vi "camara 3.vi"() -> ()   [LabVIEW 2010]
uses:
  <vilib>/addons/PixeLINK/Low Level Functions/CAMERA_FEATURES.llb/TDPU-CameraFeatures-PixelFormat.ctl
  <vilib>/Utility/error.llb/DialogType.ctl
  <vilib>/vision/Image Controls.llb/IMAQ Image.ctl
  <vilib>/addons/PixeLINK/Low Level Functions/ACQUISITION.llb/TDPU-Acquisition-StreamState.ctl
  <vilib>/addons/PixeLINK/Low Level Functions/CAMERA_FEATURES.llb/TDPU-CameraFeatures-FeatureFlags.ctl
  <vilib>/addons/PixeLINK/Low Level Functions/CAMERA_FEATURES.llb/TDPU-CameraFeatures-FeatureIds.ctl
  <vilib>/DAQmx/create/channels.llb/DAQmx Create Channel (AO-Voltage-Basic).vi
  <vilib>/DAQmx/configure/timing.llb/DAQmx Timing (Use Waveform).vi
panel:
  in  "DAQ Fs (S/s)":dbl=10000.0
  in  "Maximum Value":dbl=10.0 format="%0.2f"
  in  "Minimum Value":dbl=-10.0 format="%0.2f"
  in  "Physical Channel":tag="Dev1/ao0"
  in  "Tab Control":enum32{"Camara", "Control"}(tab)
  in  "Pixel Format Requerido":T1 items=["PIXEL_FORMAT_MONO8", "PIXEL_FORMAT_MONO16", "PIXEL_FORMAT_YUV422", "PIXEL_FORMAT_BAYER8_GRBG", "PIXEL_FORMAT_BAYER16_GRBG", "PIXEL_FORMAT_RGB24", "PIXEL_FORMAT_RGB48", "PIXEL_FORMAT_BAYER8_RGGB", "PIXEL_FORMAT_BAYER8_GBRG ", "PIXEL_FORMAT_BAYER8_BGGR ", "PIXEL_FORMAT_BAYER16_RGGB ", "PIXEL_FORMAT_BAYER16_GBRG", "PIXEL_FORMAT_BAYER16_BGGR", "PIXEL_FORMAT_RGB32"]
  in  "Exposure Time (ms)":dbl(slide) scale=0.1..2000.0
  in  "Gain":dbl(slide) scale=0.0..25.0
  in  "Red":sgl(slide) scale=0.0..4.0
  in  "Green":sgl(slide) scale=0.0..4.0
  in  "Blue":sgl(slide) scale=0.0..4.0
  in  "Selector":u16(ring) items=["776002034"]
  out "Numero de Camaras":u32
  in  "Camara ON?":bool
  in  "Ajuste ON?":bool=TRUE
  in  "Control ON?":bool=TRUE
  in  "Reset Control":bool
  in  "Parametros Ajuste nm2freq":cluster{"Cruce por cero":dbl, "Pendiente":dbl}={"Cruce por cero"=0.04, "Pendiente"=0.0031}
  in  "Frecuencia":dbl=2000.0
  in  "lamda (nm)":dbl=546.1
  out "Contraste":dbl(graph)
  out "Señal de Control":cluster{dbl[], "Señal de Control":dbl[]}(graph)
  out "Waveform":waveform(dbl)(graph)
  out "Image":T2(plugin-control)
  in  "Stop App":bool
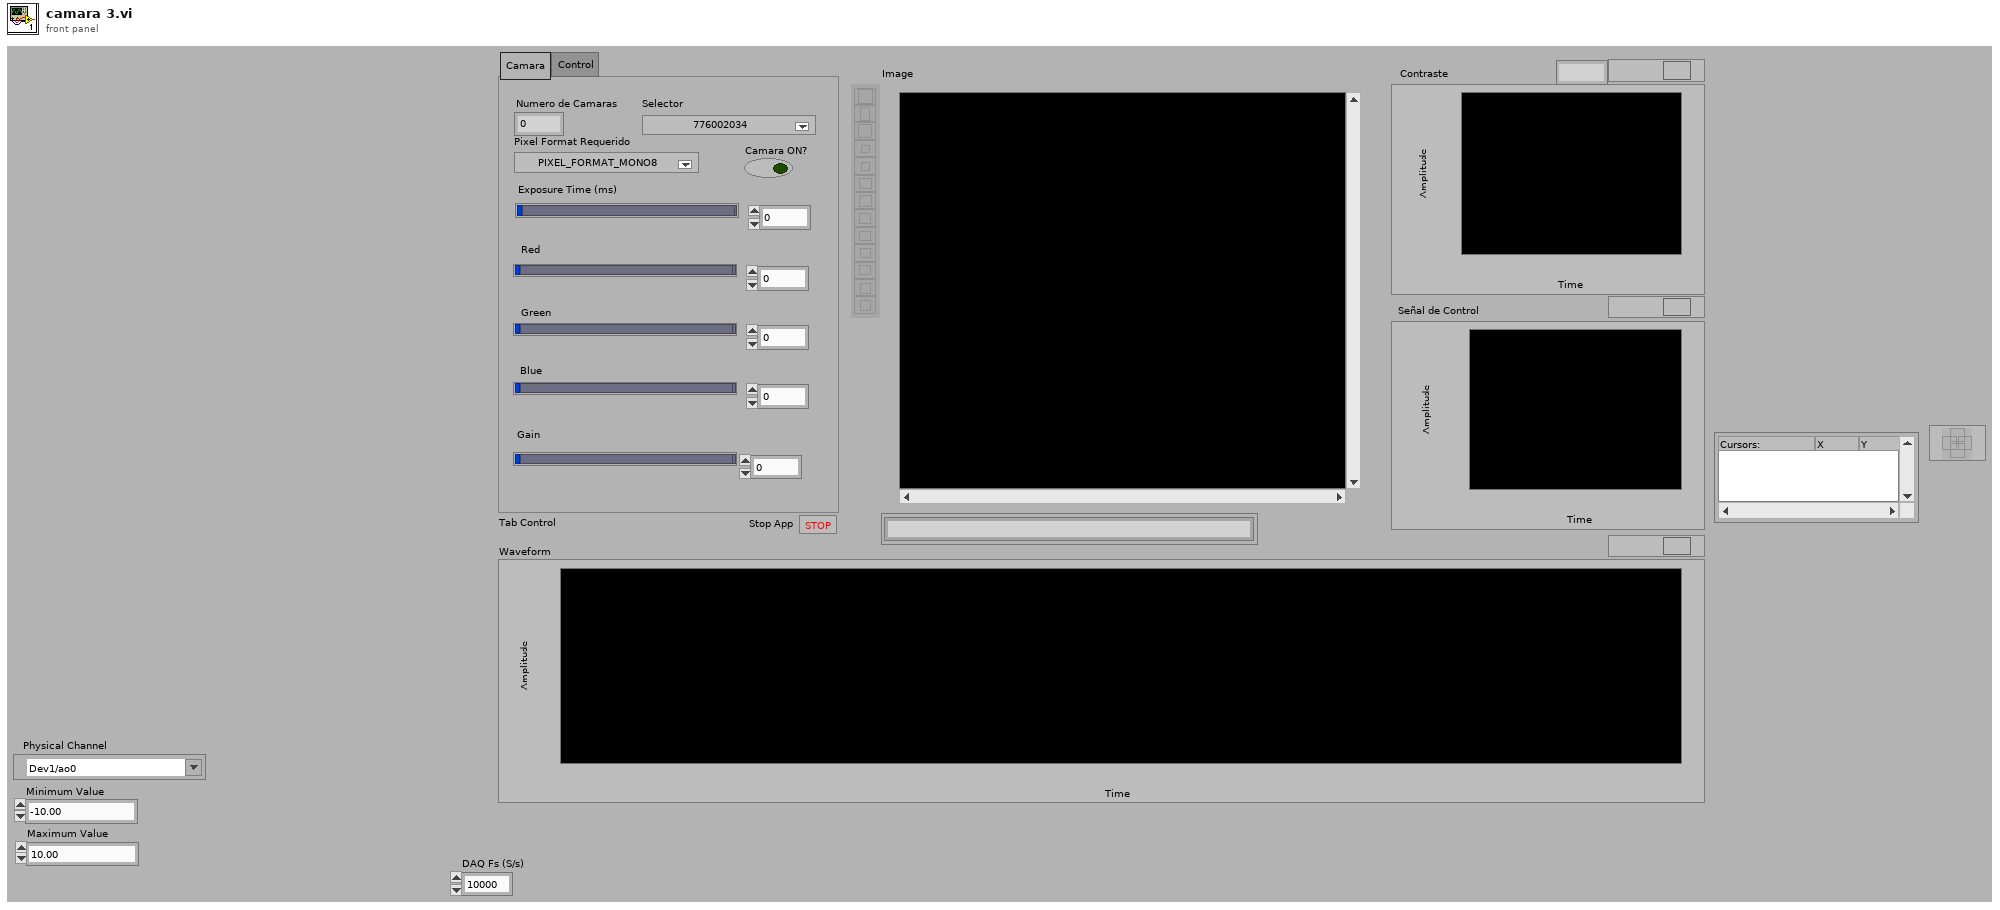
[diagram p1: front panel]
types:
  T1 = typedef "TDPU-CameraFeatures-PixelFormat.ctl" = u16
  T2 = typedef "IMAQ Image.ctl" = refnum<image>
  T3 = cluster{"DAQ Fs (S/s)":dbl, "task":refnum<k21>, "error":errorcluster}
  T4 = cluster{"lamda (nm)":dbl, "Base frecuency":dbl, "Parametros Ajuste nm2freq":cluster{"Cruce por cero":dbl, "Pendiente":dbl}}
  T5 = cluster{"Amplitud":dbl, "Media":dbl, "Sigma":dbl}
  T6 = cluster{"hCamera":u32, "errorCamera":errorcluster}
  T7 = typedef "DialogType.ctl" = u16
  T8 = typedef "Image Type" = u32
  T9 = typedef "TDPU-Acquisition-StreamState.ctl" = u32
  T10 = typedef "TDPU-CameraFeatures-FeatureIds.ctl" = u32
  T11 = typedef "TDPU-CameraFeatures-FeatureFlags.ctl" = u32
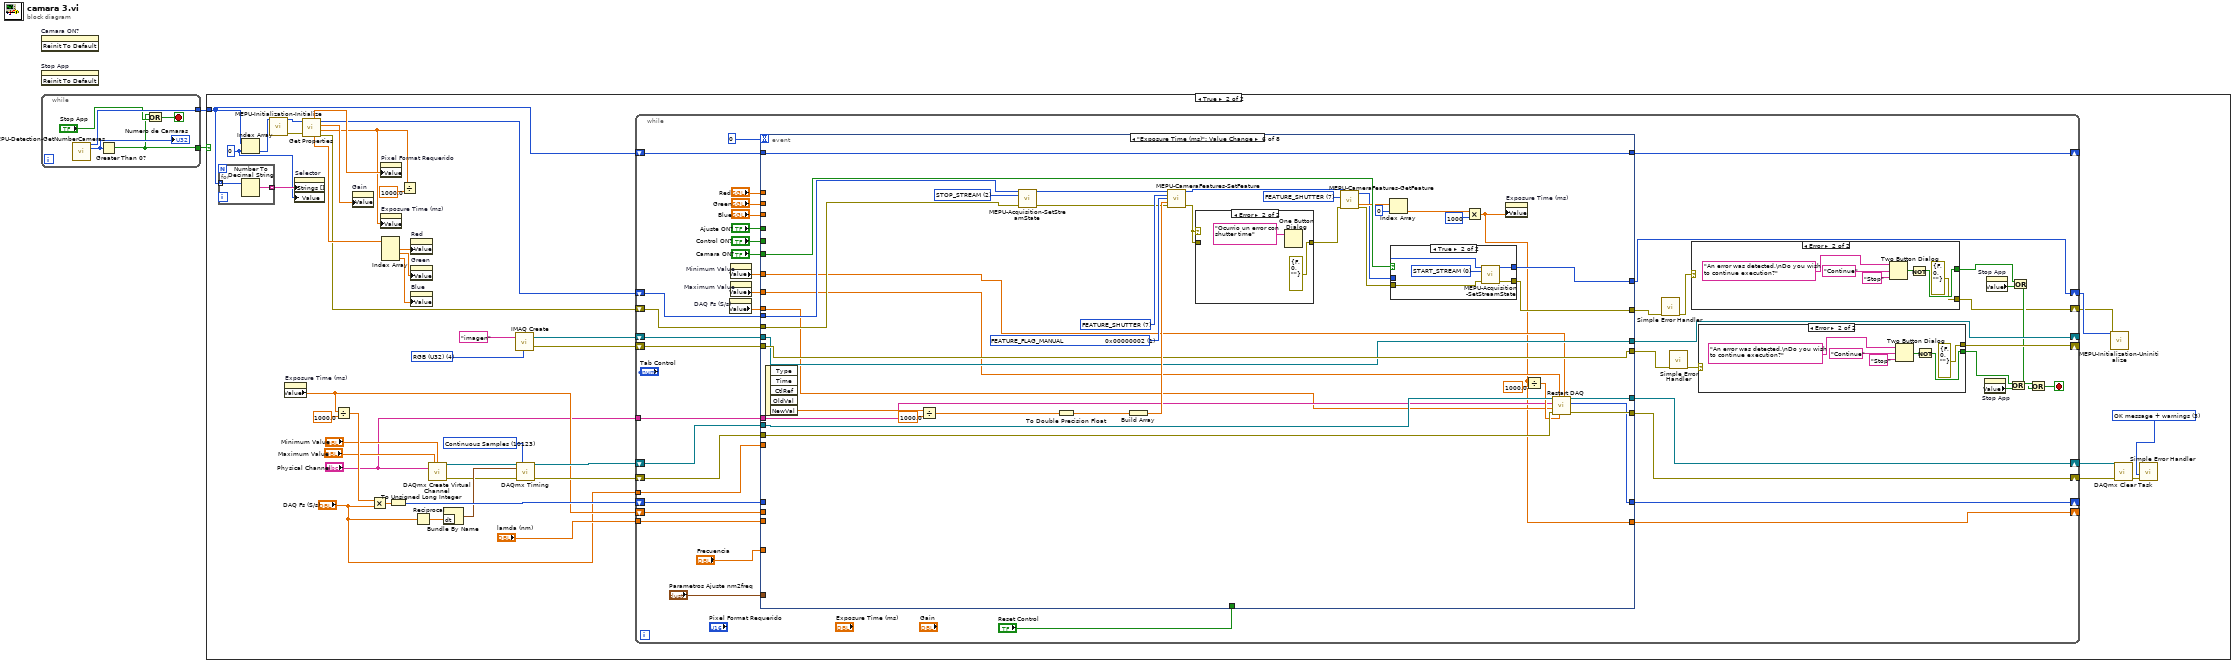
[diagram p0: block diagram]
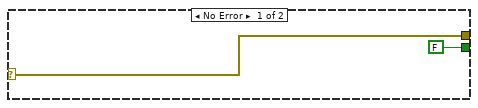
[diagram p3: hidden frame]
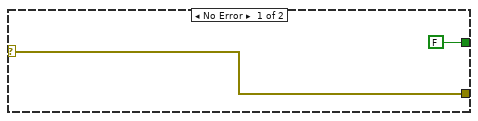
[diagram p4: hidden frame]
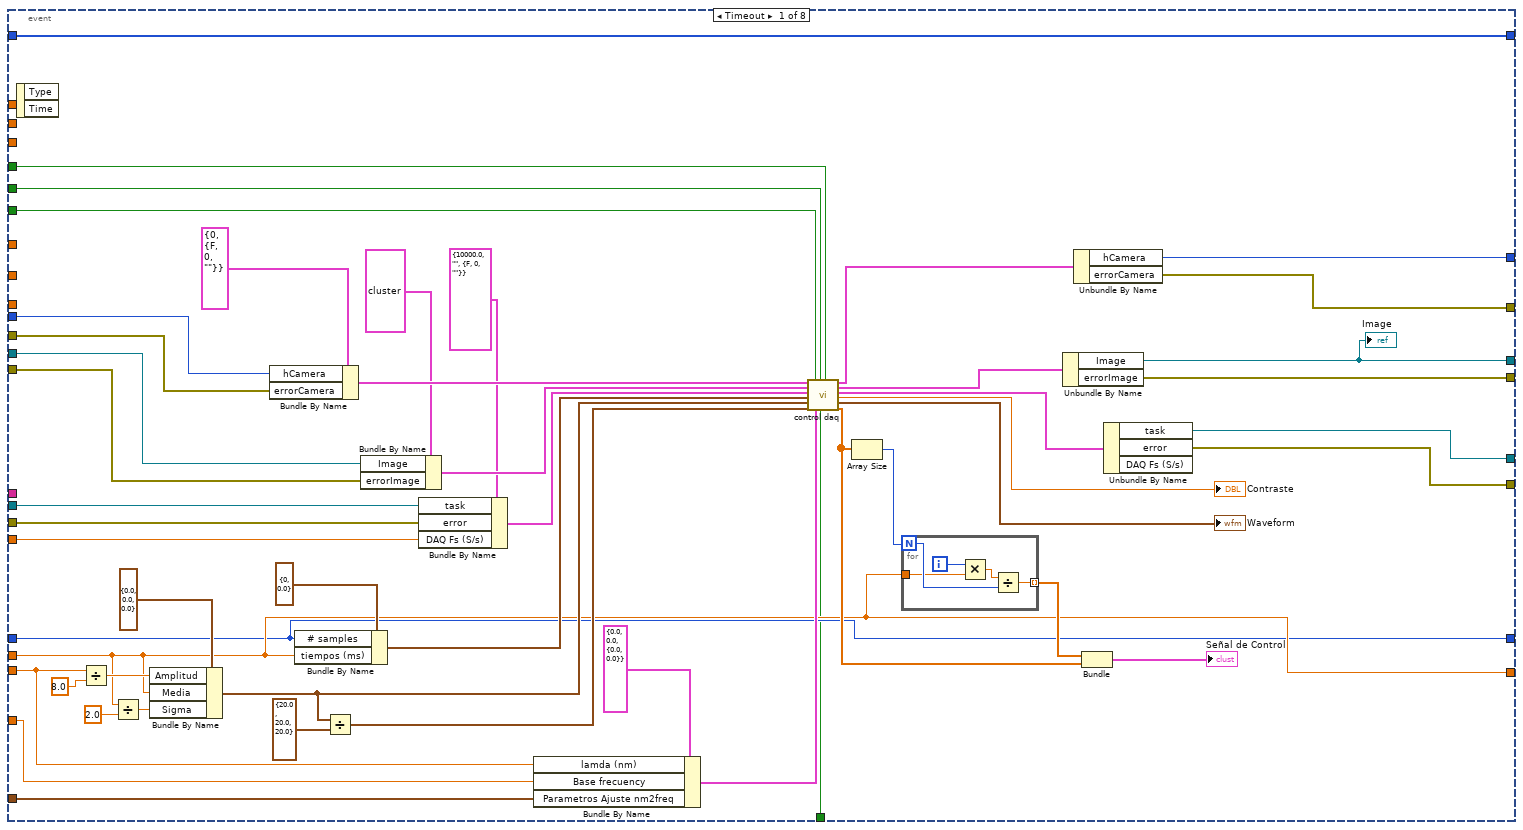
[diagram p5: hidden frame]
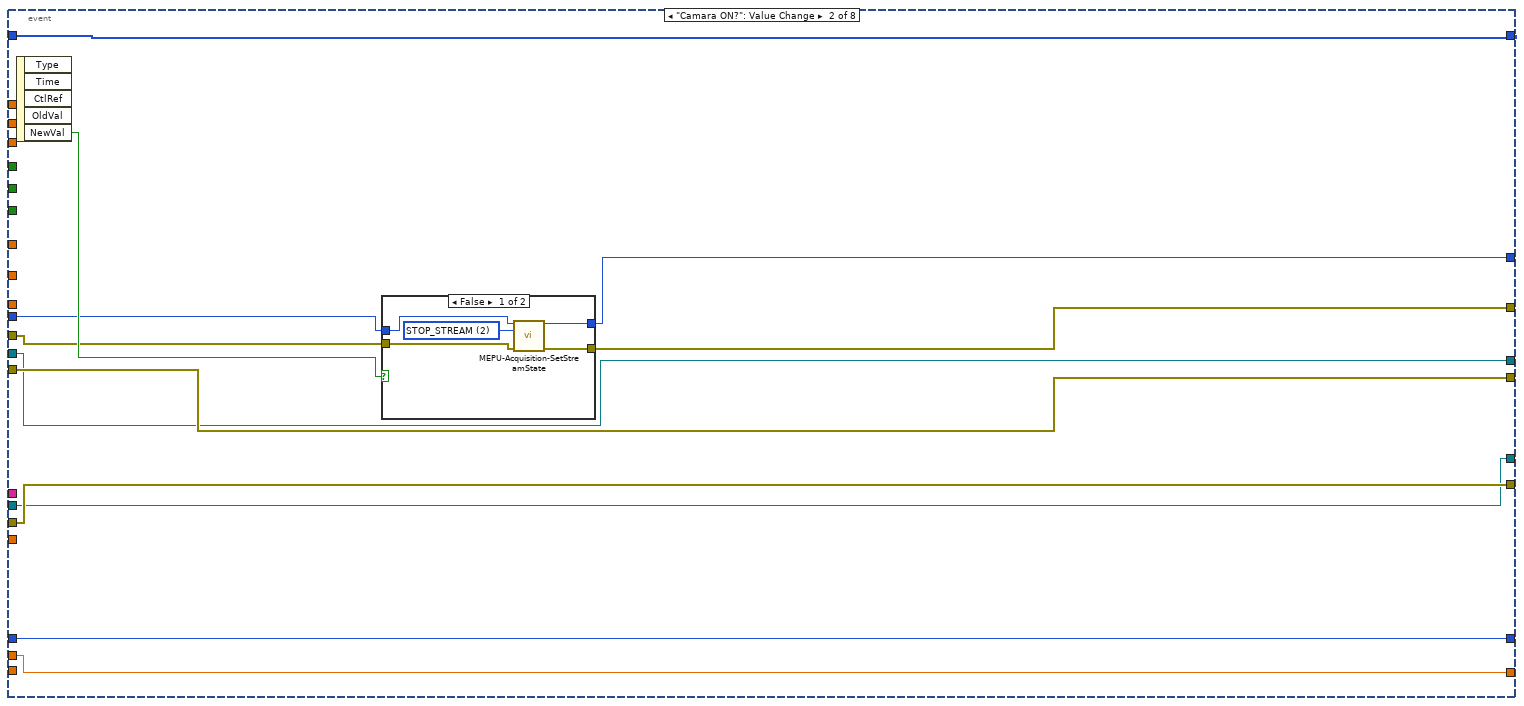
[diagram p6: hidden frame]
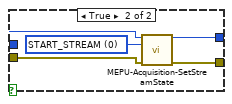
[diagram p7: hidden frame]
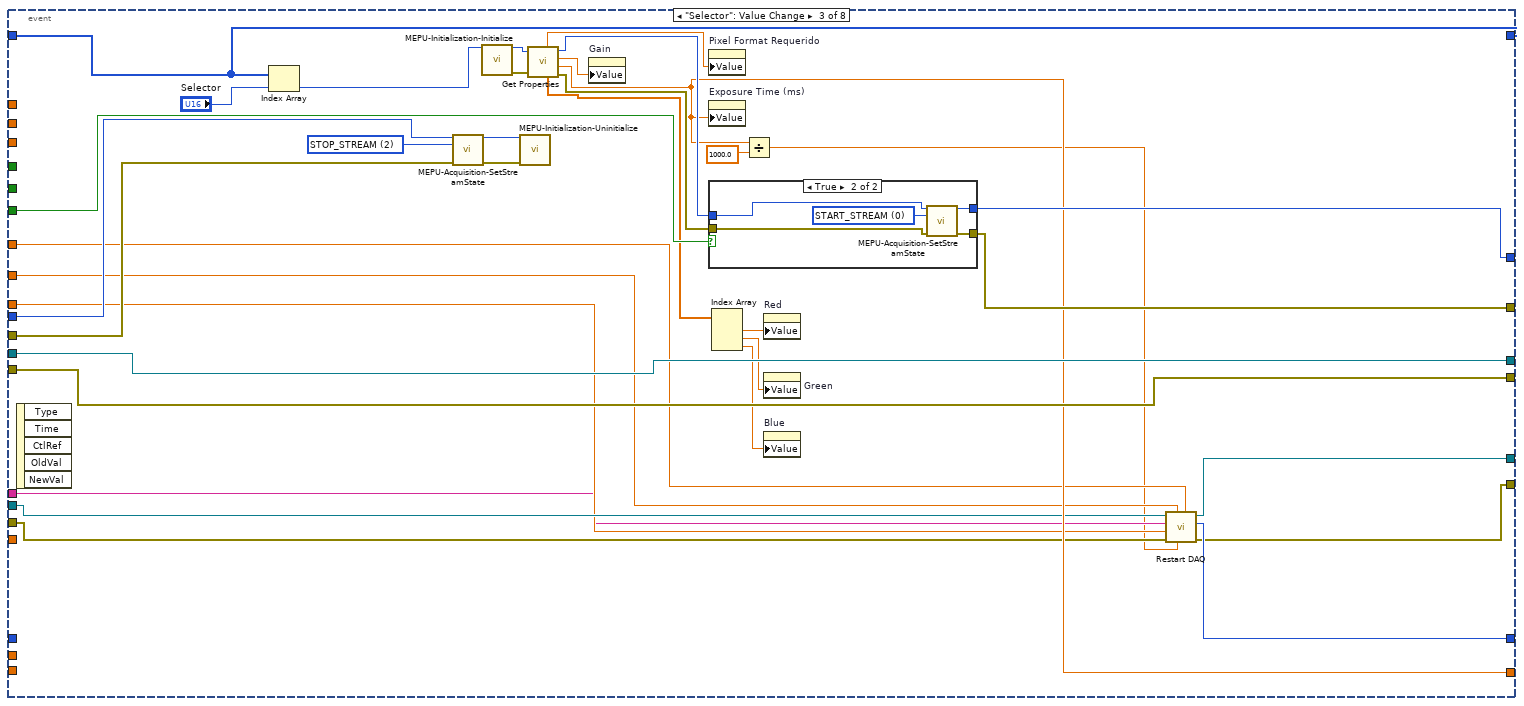
[diagram p8: hidden frame]
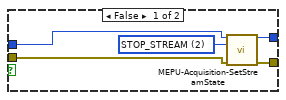
[diagram p9: hidden frame]
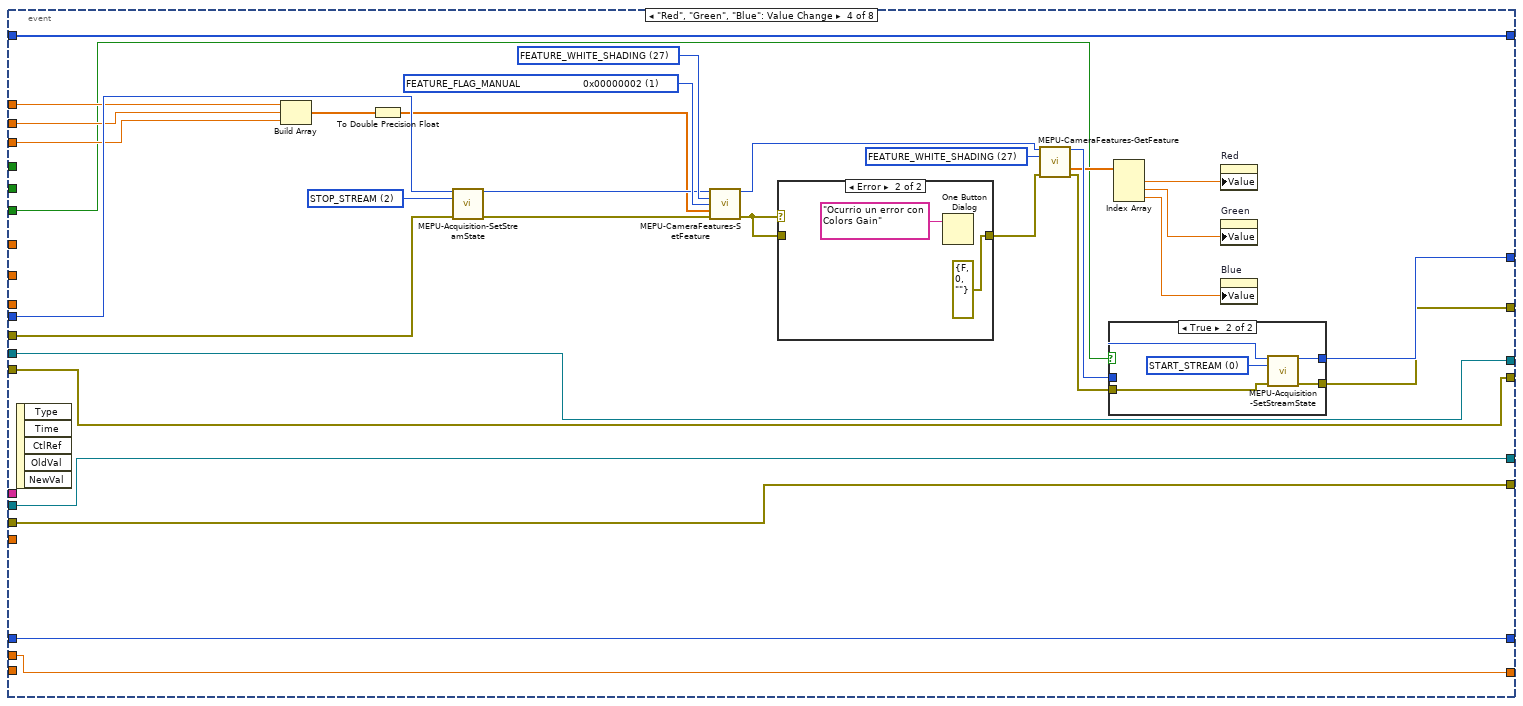
[diagram p10: hidden frame]
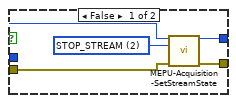
[diagram p11: hidden frame]
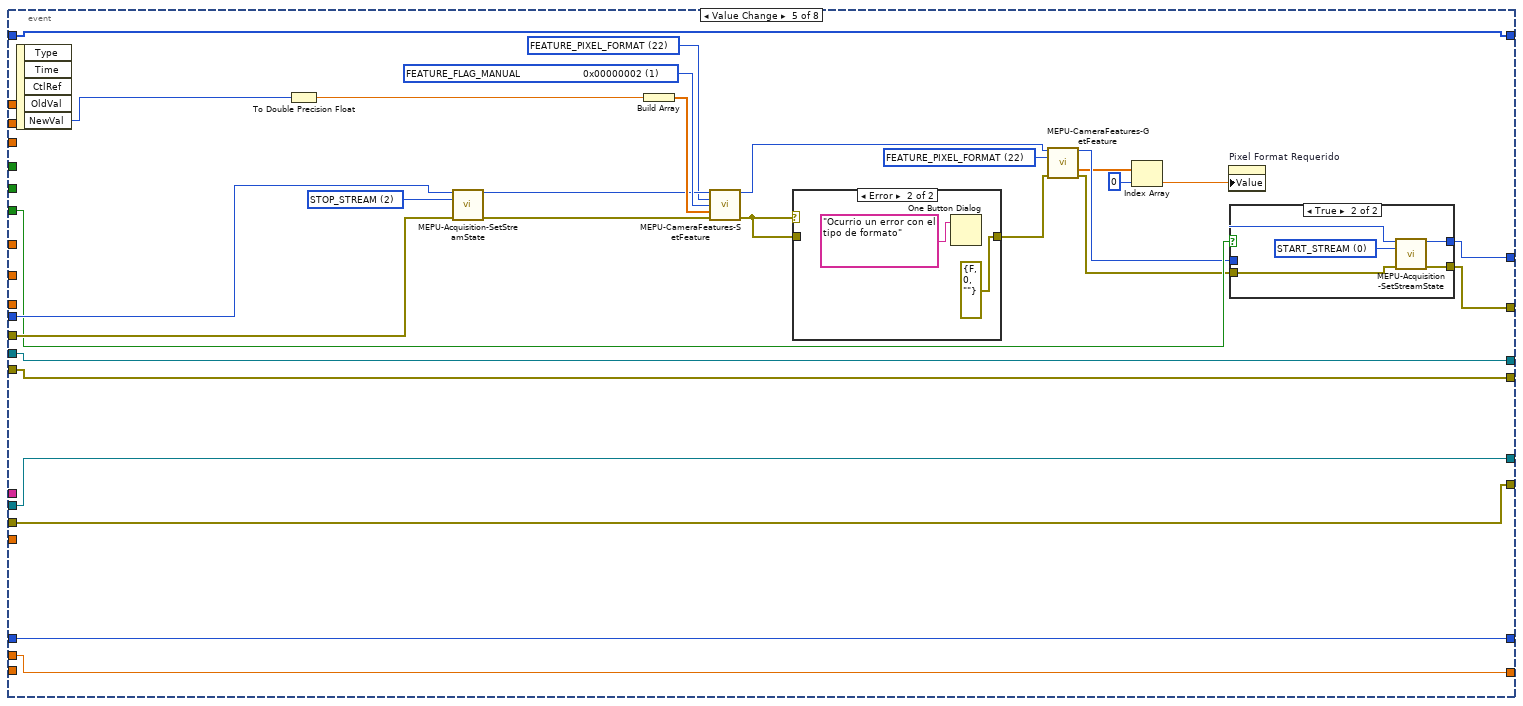
[diagram p13: hidden frame]
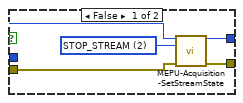
[diagram p14: hidden frame]
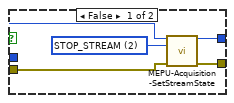
[diagram p16: hidden frame]
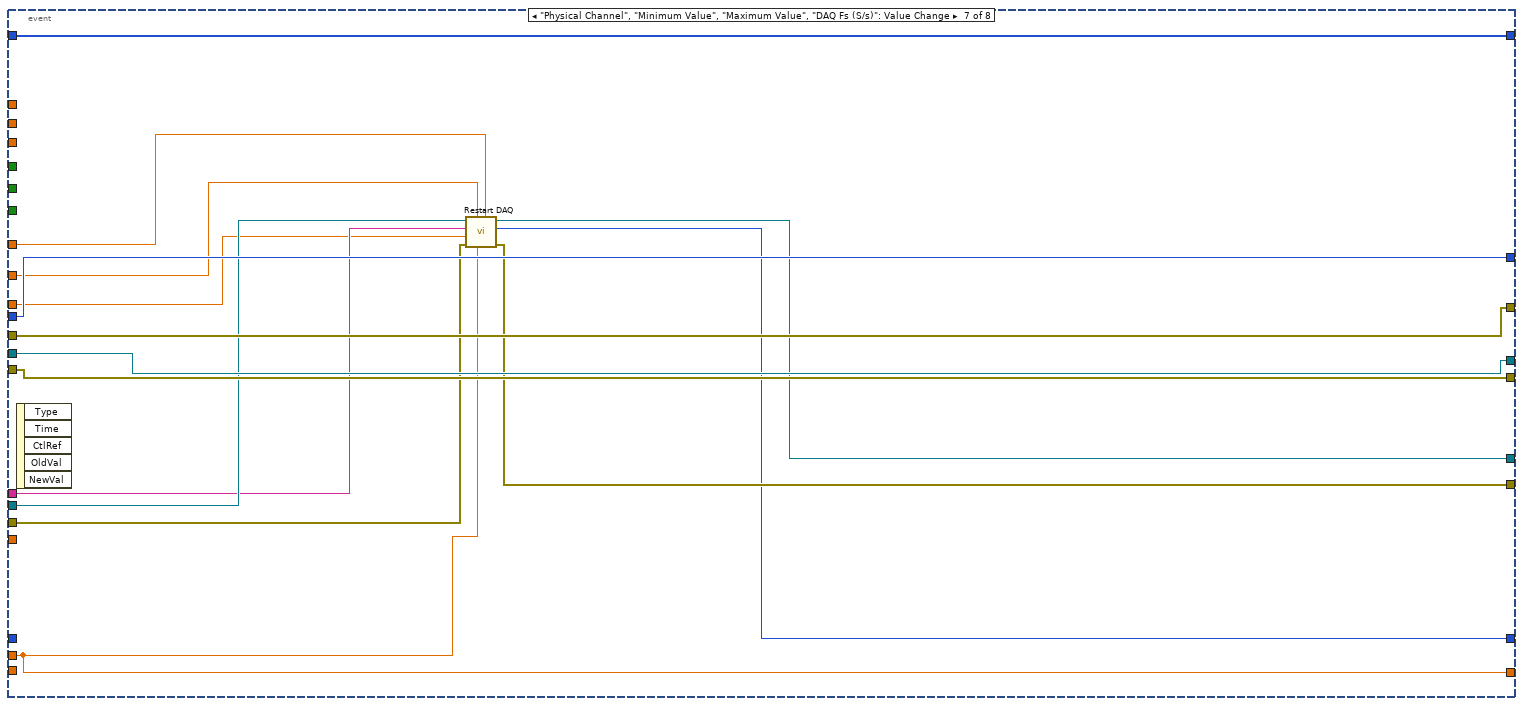
[diagram p18: hidden frame]
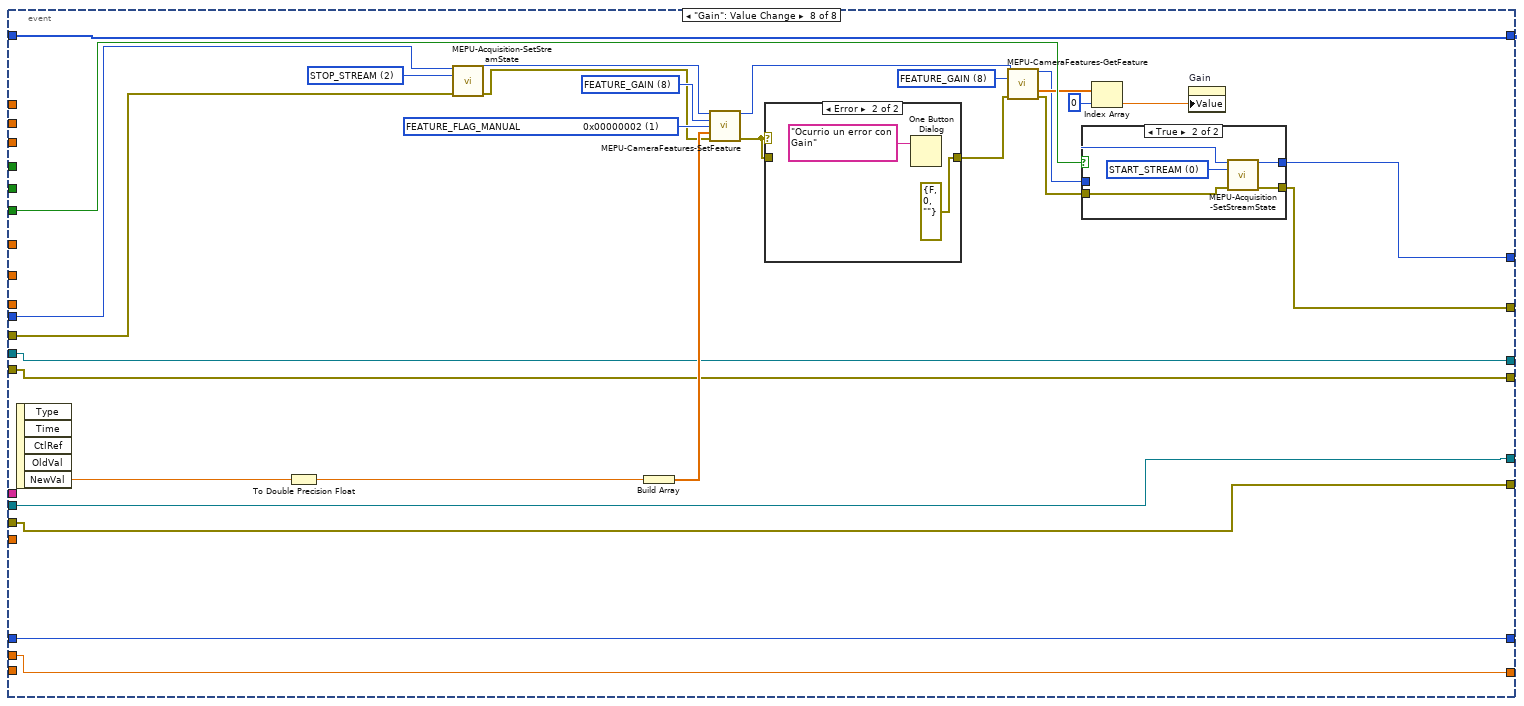
[diagram p19: hidden frame]
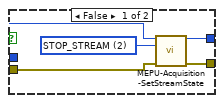
[diagram p20: hidden frame]
diagram:
  n1 = invoke on="Camara ON?" class="Bool (strict)" method="Reinit To Default"() -> ()  [unwired: 3 in, 3 out]
  n2 = invoke on="Stop App" class="Bool (strict)" method="Reinit To Default"() -> ()  [unwired: 3 in, 3 out]
  n3 = while {
    tunnel: [w7] -> w2
    tunnel: [w3] -> w1
    stop <- w5 stop-if-true
    n4 = call <vilib>:"MEPU-Detection-GetNumberCameras.vi"() -> ("LV_SerialNumbers OUT"=w7:u32[], "LV_NumberSerial OUT"=w4:u32)  [unwired: 13 in, 1 out]
    "Numero de Camaras" <- w4
    n5 = Greater Than 0?(x=w4) -> (x > 0?=w3:bool)
    n6 = Or(x=w3, y="Stop App") -> (x .or. y?=w5:bool)
  }
  n7 = case shown="True" w1 {
    tunnel: w2 -> [_ w48]
    frame False {
    }
    frame True {
      w11 = T7 3 items=["no dialog", "OK message", "continue or stop message", "OK message + warnings", "continue/stop + warnings"] ("type of dialog (OK msg:1)")
      w21 = 10123 items=["Finite Samples"=10178, "Continuous Samples"=10123, "Hardware Timed Single Point"=12522] ("sample mode")
      w42 = T8 4 items=["Grayscale (U8)", "Grayscale (I16)", "Grayscale (SGL)", "Complex (CSG)", "RGB (U32)", "HSL (U32)", "RGB (U64)", "Grayscale (U16)"] ("Image Type")
      w47 = 0
      n8 = for {
        tunnel: w48 -> [w432] mode=indexing
        tunnel: [w431] -> w50 mode=indexing
        n9 = Number To Decimal String(number=w432) -> (decimal integer string=w431:string)  [unwired: 1 in]
      }
      n10 = Index Array(array=w48, index=w47) -> (element=w49:u32)
      n11 = call <vilib>:"MEPU-Initialization-Initialize.vi"("uSerialNumber IN"=w49) -> ("phCamera OUT"=w41:u32, "Error OUT"=w40:errorcluster)  [unwired: 12 in, 1 out]
      n12 = property on="Exposure Time (ms)" class="Slide (strict)"() -> ("Value"=w14:dbl)  [unwired: 2 in, 2 out]
      n13 = property on="Selector" class="Ring (strict)"("Strings []"=w50, "Value"=w47) -> ()  [unwired: 2 in, 2 out]
      n14 = call "Get Properties.vi"("hCamera IN"=w41, "Error IN"=w40) -> ("Pixel Format OUT"=w39:dbl, "hCamera OUT"=w25:u32, "Gain OUT"=w38:dbl, "Colors Gain OUT"=w34:dbl[], "Shutter Time OUT (ms)"=w31:dbl, "Error OUT"=w24:errorcluster)  [unwired: 3 in]
      n15 = Divide(x=w14, y=sgl 1000.0) -> (x/y=w27:dbl)
      n16 = property on="Gain" class="Slide (strict)"("Value"=w38) -> ()  [unwired: 2 in, 2 out]
      n17 = Multiply(x=w27, y="DAQ Fs (S/s)") -> (x*y=w33:dbl)
      n18 = property on="Pixel Format Requerido" class="Ring (strict)"("Value"=w39) -> ()  [unwired: 2 in, 2 out]
      n19 = property on="Exposure Time (ms)" class="Slide (strict)"("Value"=w31) -> ()  [unwired: 2 in, 2 out]
      n20 = Index Array(array=w34) -> (element #1=w37:dbl, element #2=w36:dbl, element #3=w35:dbl)  [unwired: 3 in]
      n21 = To Unsigned Long Integer(number=w33) -> (unsigned 32bit integer=w29:u32)
      n22 = Divide(x=w31, y=sgl 1000.0) -> ()  [unwired: 1 out]
      n23 = property on="Red" class="Slide (strict)"("Value"=w37) -> ()  [unwired: 2 in, 2 out]
      n24 = property on="Green" class="Slide (strict)"("Value"=w36) -> ()  [unwired: 2 in, 2 out]
      n25 = property on="Blue" class="Slide (strict)"("Value"=w35) -> ()  [unwired: 2 in, 2 out]
      n26 = Reciprocal(x="DAQ Fs (S/s)") -> (1/x=w19:dbl)
      n27 = call-poly <vilib>:"DAQmx Create Virtual Channel.vi"("maximum value"="Maximum Value", "minimum value"="Minimum Value", "physical channels"="Physical Channel") -> ("task out"=w18:refnum<k21>, "error out"=w17:errorcluster)  [unwired: 11 in]
      n28 = Bundle By Name("dt"=w19) -> (w20:waveform(dbl))  [unwired: 1 in]
      n29 = call "IMAQ Create"("Image Name"="imagen", "Image Type"=w42) -> ("New Image"=w45:T2, "error out"=w43:errorcluster)  [unwired: 3 in]
      n30 = call-poly <vilib>:"DAQmx Timing.vi"("task/channels in"=w18, "sample mode"=w21, "waveform"=w20, "error in"=w17) -> ("task out"=w16:refnum<k21>, "error out"=w15:errorcluster)  [unwired: 10 in]
      n31 = while {
        shift-right: [w94] -> _
        shift-left: w48 -> [w95]
        shift-right: [w65] -> w46
        shift-left: w25 -> [w93]
        shift-right: [w64] -> w30
        shift-left: w24 -> [w92]
        shift-right: [w72] -> _
        shift-left: w43 -> [w79]
        shift-right: [w78] -> _
        shift-left: w45 -> [w85]
        shift-right: [w74] -> _
        shift-left: w14 -> [w68]
        tunnel: "lamda (nm)" -> [w67]
        shift-right: [w61] -> _
        shift-left: w29 -> [w71]
        shift-right: [w56] -> w10
        shift-left: w16 -> [w58]
        shift-right: [w55] -> w9
        shift-left: w15 -> [w57]
        tunnel: "DAQ Fs (S/s)" -> [w59]
        tunnel: "Physical Channel" -> [w54]
        stop <- w81 stop-if-true
        n32 = property on="DAQ Fs (S/s)" class="DigNum (strict)"() -> ("Value"=w51:dbl)  [unwired: 2 in, 2 out]
        n33 = property on="Minimum Value" class="DigNum (strict)"() -> ("Value"=w53:dbl)  [unwired: 2 in, 2 out]
        n34 = property on="Maximum Value" class="DigNum (strict)"() -> ("Value"=w52:dbl)  [unwired: 2 in, 2 out]
        n35 = event shown="[5] \"Exposure Time (ms)\": Value Change" {
          selector: _ -> [_ _ _ _ _ _ _ _]
          dyn-events: _ -> [_ _ _ _ _ _ _ _]
          timeout: 0 -> [_ _ _ _ _ _ _ _]
          tunnel: w95 -> [w161 w175 w221 w265 w299 w352 w388 w409]
          tunnel: [w133 w173 w214 w249 w298 w351 w384 w408] -> w65
          tunnel: [w132 w172 w215 w248 w297 w350 w385 w407] -> w87
          tunnel: [w161 w175 w221 w265 w299 w352 w388 w409] -> w94
          tunnel: w93 -> [w158 w171 w216 w251 w304 w349 w384 w406]
          tunnel: w92 -> [w157 w170 w217 w250 w303 w348 w385 w405]
          tunnel: "Camara ON?" -> [w152 _ w213 w238 w296 w347 _ w404]
          tunnel: w85 -> [w154 w176 w211 w253 w284 w333 w386 w395]
          tunnel: w79 -> [w153 w177 w212 w252 w295 w344 w387 w403]
          tunnel: [w130 w177 w212 w252 w295 w344 w387 w403] -> w84
          tunnel: [w126 w176 w211 w253 w284 w333 w386 w395] -> w78
          tunnel: "Red" -> [_ _ _ w243 _ _ _ _]
          tunnel: "Green" -> [_ _ _ w242 _ _ _ _]
          tunnel: "Blue" -> [_ _ _ w241 _ _ _ _]
          tunnel: [w128 w167 w196 w235 w279 w331 w381 w390] -> w56
          tunnel: [w127 w168 w197 w234 w280 w330 w378 w389] -> w55
          tunnel: w68 -> [w119 w174 _ w237 w282 _ w379 w392]
          tunnel: [w119 w174 w199 w237 w282 w321 w379 w392] -> w74
          tunnel: "Frecuencia" -> [w137 _ _ _ _ _ _ _]
          tunnel: w71 -> [w118 w169 _ w236 w281 _ _ w391]
          tunnel: w67 -> [w138 _ _ _ _ _ _ _]
          tunnel: "Parametros Ajuste nm2freq" -> [w136 _ _ _ _ _ _ _]
          tunnel: "Control ON?" -> [w151 _ _ _ _ _ _ _]
          tunnel: "Ajuste ON?" -> [w150 _ _ _ _ _ _ _]
          tunnel: [w118 w169 w198 w236 w281 w329 w377 w391] -> w61
          tunnel: "Reset Control" -> [w117 _ _ _ _ _ _ _]
          tunnel: w59 -> [w114 _ _ _ _ _ _ _]
          tunnel: w58 -> [w113 w167 w193 w235 w279 w328 w383 w390]
          tunnel: w57 -> [w112 w168 w192 w234 w280 w327 w382 w389]
          tunnel: w54 -> [_ _ w190 _ _ w323 w380 _]
          tunnel: w53 -> [_ _ w195 _ _ w324 w376 _]
          tunnel: w52 -> [_ _ w194 _ _ w325 w375 _]
          tunnel: w51 -> [_ _ w191 _ _ w322 w374 _]
          event Timeout {
            n36 = event-data() -> ()  [unwired: 1 in, 2 out]
            n37 = Divide(x=w138, y=8.0) -> (x/y=w143:dbl)
            n38 = Divide(x=w119, y=2.0) -> (x/y=w146:dbl)
            n39 = Bundle By Name(cluster=T5 {"Amplitud"=0.0, "Media"=0.0, "Sigma"=0.0} ("Parametros Maximos"), "Amplitud"=w143, "Media"=w119, "Sigma"=w146) -> (w141:T5)
            n40 = Bundle By Name(cluster=T6 {"hCamera"=0, "errorCamera"={"status"=FALSE, "code"=0, "source"=""}} ("Camera Device IN"), "hCamera"=w158, "errorCamera"=w157) -> (w159:T6)
            n41 = Bundle By Name(cluster=cluster{"# samples":u32, "tiempos (ms)":dbl} {"# samples"=0, "tiempos (ms)"=0.0} ("Sound Parameters"), "# samples"=w118, "tiempos (ms)"=w119) -> (w148:cluster{"# samples":u32, "tiempos (ms)":dbl})
            n42 = Divide(x=w141, y=T5 {"Amplitud"=20.0, "Media"=20.0, "Sigma"=20.0}) -> (x/y=w140:T5)
            n43 = Bundle By Name(cluster=cluster{"Image":T2, "errorImage":errorcluster} {"Image"=refnum, "errorImage"={"status"=FALSE, "code"=0, "source"=""}} ("Image Device IN"), "Image"=w154, "errorImage"=w153) -> (w155:cluster{"Image":T2, "errorImage":errorcluster})
            n44 = Bundle By Name(cluster=T3 {"DAQ Fs (S/s)"=10000.0, "task"="", "error"={"status"=FALSE, "code"=0, "source"=""}} ("DAQ Device IN"), "task"=w113, "error"=w112, "DAQ Fs (S/s)"=w114) -> (w115:T3)
            n45 = Bundle By Name(cluster=T4 {"lamda (nm)"=0.0, "Base frecuency"=0.0, "Parametros Ajuste nm2freq"={"Cruce por cero"=0.0, "Pendiente"=0.0}} ("Parametros Interferometro/Freq-Volt"), "lamda (nm)"=w138, "Base frecuency"=w137, "Parametros Ajuste nm2freq"=w136) -> (w135:T4)
            n46 = call "control daq.vi"("Camera Device IN"=w159, "Image Device IN"=w155, "DAQ Device IN"=w115, "Time Control Parameters"=w148, "Parametros Maximos"=w141, "detla Parametros"=w140, "Camara ON?"=w152, "Parametros Interferometro/Freq-Volt"=w135, "Control?"=w151, "Reset Control"=w117, "Ajuste?"=w150) -> ("Camara Device OUT"=w134:T6, "Image Device OUT"=w131:cluster{"Image":T2, "errorImage":errorcluster}, "DAQ Device OUT"=w129:T3, "Contraste"=→"Contraste":dbl, "Waveform"=→"Waveform":waveform(dbl), "Señal de Control"=w121:dbl[])  [unwired: 3 in]
            n47 = Array Size(array=w121) -> (size(s)=w124:i32)
            n48 = for {
              N: w124 -> [w163]
              tunnel: [w164] -> w122 mode=indexing
              tunnel: w119 -> [w162]
              i -> [w166]
              n49 = Multiply(x=w166, y=w162) -> (x*y=w165:dbl)
              n50 = Divide(x=w165, y=w163) -> (x/y=w164:dbl)
            }
            n51 = Unbundle By Name(w131) -> ("Image"=w126:T2, "errorImage"=w130:errorcluster)
            "Image" <- w126
            n52 = Unbundle By Name(w134) -> ("hCamera"=w133:u32, "errorCamera"=w132:errorcluster)
            n53 = Bundle(w122, "Señal de Control"=w121) -> (→"Señal de Control":cluster{dbl[], "Señal de Control":dbl[]})  [unwired: 1 in]
            n54 = Unbundle By Name(w129) -> ("task"=w128:refnum<k21>, "error"=w127:errorcluster)  [unwired: 1 out]
          }
          event "Camara ON?": Value Change {
            n55 = event-data() -> ("NewVal"=w178:bool)  [unwired: 1 in, 4 out]
            n56 = case shown="False" w178 {
              tunnel: w171 -> [w179 w187]
              tunnel: w170 -> [w182 w186]
              tunnel: [w180 w185] -> w172
              tunnel: [w181 w184] -> w173
              frame False {
                w183 = T9 2 items=["START_STREAM", "PAUSE_STREAM", "STOP_STREAM"] ("uStreamState IN")
                n57 = call <vilib>:"MEPU-Acquisition-SetStreamState.vi"("hCamera IN"=w179, "uStreamState IN"=w183, "Error IN"=w182) -> ("hCamera OUT"=w181:u32, "Error OUT"=w180:errorcluster)  [unwired: 11 in]
              }
              frame True {
                w188 = T9 0 items=["START_STREAM", "PAUSE_STREAM", "STOP_STREAM"] ("uStreamState IN")
                n58 = call <vilib>:"MEPU-Acquisition-SetStreamState.vi"("hCamera IN"=w187, "uStreamState IN"=w188, "Error IN"=w186) -> ("hCamera OUT"=w184:u32, "Error OUT"=w185:errorcluster)  [unwired: 11 in]
              }
            }
          }
          event "Selector": Value Change {
            w220 = T9 2 items=["START_STREAM", "PAUSE_STREAM", "STOP_STREAM"] ("uStreamState IN")
            n59 = event-data() -> ()  [unwired: 1 in, 5 out]
            n60 = Index Array(array=w221, index="Selector") -> (element=w222:u32)
            n61 = call <vilib>:"MEPU-Acquisition-SetStreamState.vi"("hCamera IN"=w216, "uStreamState IN"=w220, "Error IN"=w217) -> ("hCamera OUT"=w218:u32, "Error OUT"=w219:errorcluster)  [unwired: 11 in]
            n62 = call <vilib>:"MEPU-Initialization-Initialize.vi"("uSerialNumber IN"=w222) -> ("phCamera OUT"=w207:u32, "Error OUT"=w206:errorcluster)  [unwired: 12 in, 1 out]
            n63 = call <vilib>:"MEPU-Initialization-Uninitialize.vi"("hCamera IN"=w218, "Error IN"=w219) -> ()  [unwired: 13 in, 1 out]
            n64 = call "Get Properties.vi"("hCamera IN"=w207, "Error IN"=w206) -> ("Pixel Format OUT"=w205:dbl, "hCamera OUT"=w203:u32, "Gain OUT"=w202:dbl, "Colors Gain OUT"=w201:dbl[], "Shutter Time OUT (ms)"=w199:dbl, "Error OUT"=w204:errorcluster)  [unwired: 3 in]
            n65 = property on="Gain" class="Slide (strict)"("Value"=w202) -> ()  [unwired: 2 in, 2 out]
            n66 = property on="Pixel Format Requerido" class="Ring (strict)"("Value"=w205) -> ()  [unwired: 2 in, 2 out]
            n67 = property on="Exposure Time (ms)" class="Slide (strict)"("Value"=w199) -> ()  [unwired: 2 in, 2 out]
            n68 = case shown="True" w213 {
              tunnel: [w226 w232] -> w215
              tunnel: [w227 w231] -> w214
              tunnel: w204 -> [w225 w230]
              tunnel: w203 -> [w224 w229]
              frame False {
                w228 = T9 2 items=["START_STREAM", "PAUSE_STREAM", "STOP_STREAM"] ("uStreamState IN")
                n69 = call <vilib>:"MEPU-Acquisition-SetStreamState.vi"("hCamera IN"=w224, "uStreamState IN"=w228, "Error IN"=w225) -> ("hCamera OUT"=w227:u32, "Error OUT"=w226:errorcluster)  [unwired: 11 in]
              }
              frame True {
                w233 = T9 0 items=["START_STREAM", "PAUSE_STREAM", "STOP_STREAM"] ("uStreamState IN")
                n70 = call <vilib>:"MEPU-Acquisition-SetStreamState.vi"("hCamera IN"=w229, "uStreamState IN"=w233, "Error IN"=w230) -> ("hCamera OUT"=w231:u32, "Error OUT"=w232:errorcluster)  [unwired: 11 in]
              }
            }
            n71 = Index Array(array=w201) -> (element #1=w210:dbl, element #2=w209:dbl, element #3=w208:dbl)  [unwired: 3 in]
            n72 = Divide(x=w199, y=sgl 1000.0) -> (x/y=w189:dbl)
            n73 = property on="Red" class="Slide (strict)"("Value"=w210) -> ()  [unwired: 2 in, 2 out]
            n74 = property on="Green" class="Slide (strict)"("Value"=w209) -> ()  [unwired: 2 in, 2 out]
            n75 = property on="Blue" class="Slide (strict)"("Value"=w208) -> ()  [unwired: 2 in, 2 out]
            n76 = call "Restart DAQ.vi"("Min Value"=w195, "tiempo (s)"=w189, "Max Value"=w194, "error IN"=w192, "Fs (S/s)"=w191, "Physical Channel"=w190, "task IN"=w193) -> ("error OUT"=w197:errorcluster, "# samples"=w198:u32, "task OUT"=w196:refnum<k21>)  [unwired: 2 in]
          }
          event "Red", "Green", "Blue": Value Change {
            w258 = T10 27 items=["FEATURE_BRIGHTNESS", "FEATURE_EXPOSURE", "FEATURE_SHARPNESS", "FEATURE_WHITE_BAL", "FEATURE_HUE", "FEATURE_SATURATION", "FEATURE_GAMMA", "FEATURE_SHUTTER", "FEATURE_GAIN", "FEATURE_IRIS", "FEATURE_FOCUS", "FEATURE_TEMPERATURE", "FEATURE_TRIGGER", "FEATURE_ZOOM", "FEATURE_PAN", "FEATURE_TILT", "FEATURE_OPT_FILTER", "FEATURE_GPIO", "FEATURE_FRAME_RATE", "FEATURE_ROI", "FEATURE_FLIP", "FEATURE_PIXEL_ADDRESSING", "FEATURE_PIXEL_FORMAT", "FEATURE_EXTENDED_SHUTTER", "FEATURE_AUTO_ROI", "FEATURE_LOOKUP_TABLE", "FEATURE_MEMORY_CHANNEL", "FEATURE_WHITE_SHADING", "FEATURE_ROTATE", "FEATURE_IMAGER_CLK_DIVISOR", "FEATURE_TRIG_WITH_CNTRLD_LIGHT", "FEATURE_MAX_PIXEL_SIZE"] ("uFeatureId IN")
            w259 = T9 2 items=["START_STREAM", "PAUSE_STREAM", "STOP_STREAM"] ("uStreamState IN")
            w263 = T11 1 items=["FEATURE_FLAG_PRESENCE                 0x00000001", "FEATURE_FLAG_MANUAL                     0x00000002", "FEATURE_FLAG_AUTO                         0x00000004", "FEATURE_FLAG_ONEPUSH                   0x00000008", "FEATURE_FLAG_OFF                            0x00000010", "FEATURE_FLAG_DESC_SUPPORTED    0x00000020", "FEATURE_FLAG_READ_ONLY               0x00000040"] ("uFlags IN")
            w264 = T10 27 items=["FEATURE_BRIGHTNESS", "FEATURE_EXPOSURE", "FEATURE_SHARPNESS", "FEATURE_WHITE_BAL", "FEATURE_HUE", "FEATURE_SATURATION", "FEATURE_GAMMA", "FEATURE_SHUTTER", "FEATURE_GAIN", "FEATURE_IRIS", "FEATURE_FOCUS", "FEATURE_TEMPERATURE", "FEATURE_TRIGGER", "FEATURE_ZOOM", "FEATURE_PAN", "FEATURE_TILT", "FEATURE_OPT_FILTER", "FEATURE_GPIO", "FEATURE_FRAME_RATE", "FEATURE_ROI", "FEATURE_FLIP", "FEATURE_PIXEL_ADDRESSING", "FEATURE_PIXEL_FORMAT", "FEATURE_EXTENDED_SHUTTER", "FEATURE_AUTO_ROI", "FEATURE_LOOKUP_TABLE", "FEATURE_MEMORY_CHANNEL", "FEATURE_WHITE_SHADING", "FEATURE_ROTATE", "FEATURE_IMAGER_CLK_DIVISOR", "FEATURE_TRIG_WITH_CNTRLD_LIGHT", "FEATURE_MAX_PIXEL_SIZE"] ("uFeatureId IN")
            n77 = event-data() -> ()  [unwired: 1 in, 5 out]
            n78 = Build Array(w243, w242, w241) -> (w240:sgl[])
            n79 = To Double Precision Float(number=w240) -> (double precision float=w239:dbl[])
            n80 = call <vilib>:"MEPU-Acquisition-SetStreamState.vi"("hCamera IN"=w251, "uStreamState IN"=w259, "Error IN"=w250) -> ("hCamera OUT"=w261:u32, "Error OUT"=w260:errorcluster)  [unwired: 11 in]
            n81 = call <vilib>:"MEPU-CameraFeatures-SetFeature.vi"("hCamera IN"=w261, "uFeatureId IN"=w264, "uFlags IN"=w263, "pParms IN"=w239, "Error IN"=w260) -> ("hCamera OUT"=w257:u32, "Error OUT"=w262:errorcluster)  [unwired: 8 in, 1 out]
            n82 = case shown="Error" w262 {
              tunnel: [w276 errorcluster {"status"=FALSE, "code"=0, "source"=""} ("Error OUT")] -> w254
              tunnel: w262 -> [w276 _]
              frame No Error {
              }
              frame Error {
                n83 = One Button Dialog(message="Ocurrio un error con Colors Gain") -> ()  [unwired: 1 in, 1 out]
              }
            }
            n84 = call <vilib>:"MEPU-CameraFeatures-GetFeature.vi"("hCamera IN"=w257, "uFeatureId IN"=w258, "Error IN"=w254) -> ("hCamera OUT"=w256:u32, "pParms OUT"=w244:dbl[], "Error OUT"=w255:errorcluster)  [unwired: 8 in, 2 out]
            n85 = case shown="True" w238 {
              tunnel: w255 -> [w269 w274]
              tunnel: [w267 w273] -> w248
              tunnel: [w268 w272] -> w249
              tunnel: w256 -> [w266 w271]
              frame False {
                w270 = T9 2 items=["START_STREAM", "PAUSE_STREAM", "STOP_STREAM"] ("uStreamState IN")
                n86 = call <vilib>:"MEPU-Acquisition-SetStreamState.vi"("hCamera IN"=w266, "uStreamState IN"=w270, "Error IN"=w269) -> ("hCamera OUT"=w268:u32, "Error OUT"=w267:errorcluster)  [unwired: 11 in]
              }
              frame True {
                w275 = T9 0 items=["START_STREAM", "PAUSE_STREAM", "STOP_STREAM"] ("uStreamState IN")
                n87 = call <vilib>:"MEPU-Acquisition-SetStreamState.vi"("hCamera IN"=w271, "uStreamState IN"=w275, "Error IN"=w274) -> ("hCamera OUT"=w272:u32, "Error OUT"=w273:errorcluster)  [unwired: 11 in]
              }
            }
            n88 = Index Array(array=w244) -> (element #1=w247:dbl, element #2=w246:dbl, element #3=w245:dbl)  [unwired: 3 in]
            n89 = property on="Red" class="Slide (strict)"("Value"=w247) -> ()  [unwired: 2 in, 2 out]
            n90 = property on="Green" class="Slide (strict)"("Value"=w246) -> ()  [unwired: 2 in, 2 out]
            n91 = property on="Blue" class="Slide (strict)"("Value"=w245) -> ()  [unwired: 2 in, 2 out]
          }
          event Value Change {
            w289 = T10 22 items=["FEATURE_BRIGHTNESS", "FEATURE_EXPOSURE", "FEATURE_SHARPNESS", "FEATURE_WHITE_BAL", "FEATURE_HUE", "FEATURE_SATURATION", "FEATURE_GAMMA", "FEATURE_SHUTTER", "FEATURE_GAIN", "FEATURE_IRIS", "FEATURE_FOCUS", "FEATURE_TEMPERATURE", "FEATURE_TRIGGER", "FEATURE_ZOOM", "FEATURE_PAN", "FEATURE_TILT", "FEATURE_OPT_FILTER", "FEATURE_GPIO", "FEATURE_FRAME_RATE", "FEATURE_ROI", "FEATURE_FLIP", "FEATURE_PIXEL_ADDRESSING", "FEATURE_PIXEL_FORMAT", "FEATURE_EXTENDED_SHUTTER", "FEATURE_AUTO_ROI", "FEATURE_LOOKUP_TABLE", "FEATURE_MEMORY_CHANNEL", "FEATURE_WHITE_SHADING", "FEATURE_ROTATE", "FEATURE_IMAGER_CLK_DIVISOR", "FEATURE_TRIG_WITH_CNTRLD_LIGHT", "FEATURE_MAX_PIXEL_SIZE"] ("uFeatureId IN")
            w300 = T9 2 items=["START_STREAM", "PAUSE_STREAM", "STOP_STREAM"] ("uStreamState IN")
            w307 = T11 1 items=["FEATURE_FLAG_PRESENCE                 0x00000001", "FEATURE_FLAG_MANUAL                     0x00000002", "FEATURE_FLAG_AUTO                         0x00000004", "FEATURE_FLAG_ONEPUSH                   0x00000008", "FEATURE_FLAG_OFF                            0x00000010", "FEATURE_FLAG_DESC_SUPPORTED    0x00000020", "FEATURE_FLAG_READ_ONLY               0x00000040"] ("uFlags IN")
            w294 = T10 22 items=["FEATURE_BRIGHTNESS", "FEATURE_EXPOSURE", "FEATURE_SHARPNESS", "FEATURE_WHITE_BAL", "FEATURE_HUE", "FEATURE_SATURATION", "FEATURE_GAMMA", "FEATURE_SHUTTER", "FEATURE_GAIN", "FEATURE_IRIS", "FEATURE_FOCUS", "FEATURE_TEMPERATURE", "FEATURE_TRIGGER", "FEATURE_ZOOM", "FEATURE_PAN", "FEATURE_TILT", "FEATURE_OPT_FILTER", "FEATURE_GPIO", "FEATURE_FRAME_RATE", "FEATURE_ROI", "FEATURE_FLIP", "FEATURE_PIXEL_ADDRESSING", "FEATURE_PIXEL_FORMAT", "FEATURE_EXTENDED_SHUTTER", "FEATURE_AUTO_ROI", "FEATURE_LOOKUP_TABLE", "FEATURE_MEMORY_CHANNEL", "FEATURE_WHITE_SHADING", "FEATURE_ROTATE", "FEATURE_IMAGER_CLK_DIVISOR", "FEATURE_TRIG_WITH_CNTRLD_LIGHT", "FEATURE_MAX_PIXEL_SIZE"] ("uFeatureId IN")
            n92 = event-data() -> ("NewVal"=w285:T1)  [unwired: 1 in, 4 out]
            n93 = To Double Precision Float(number=w285) -> (double precision float=w305:dbl)
            n94 = call <vilib>:"MEPU-Acquisition-SetStreamState.vi"("hCamera IN"=w304, "uStreamState IN"=w300, "Error IN"=w303) -> ("hCamera OUT"=w302:u32, "Error OUT"=w301:errorcluster)  [unwired: 11 in]
            n95 = Build Array(w305) -> (w306:dbl[])
            n96 = call <vilib>:"MEPU-CameraFeatures-SetFeature.vi"("hCamera IN"=w302, "uFeatureId IN"=w294, "uFlags IN"=w307, "pParms IN"=w306, "Error IN"=w301) -> ("hCamera OUT"=w291:u32, "Error OUT"=w287:errorcluster)  [unwired: 8 in, 1 out]
            n97 = case shown="Error" w287 {
              tunnel: [w318 errorcluster {"status"=FALSE, "code"=0, "source"=""} ("Error OUT")] -> w286
              tunnel: w287 -> [w318 _]
              frame No Error {
              }
              frame Error {
                n98 = One Button Dialog(message="Ocurrio un error con el tipo de formato") -> ()  [unwired: 1 in, 1 out]
              }
            }
            n99 = call <vilib>:"MEPU-CameraFeatures-GetFeature.vi"("hCamera IN"=w291, "uFeatureId IN"=w289, "Error IN"=w286) -> ("hCamera OUT"=w290:u32, "pParms OUT"=w288:dbl[], "Error OUT"=w292:errorcluster)  [unwired: 8 in, 2 out]
            n100 = Index Array(array=w288, index=0) -> (element=w283:dbl)
            n101 = property on="Pixel Format Requerido" class="Ring (strict)"("Value"=w283) -> ()  [unwired: 2 in, 2 out]
            n102 = case shown="True" w296 {
              tunnel: w290 -> [w311 w316]
              tunnel: w292 -> [w310 w315]
              tunnel: [w308 w314] -> w297
              tunnel: [w309 w313] -> w298
              frame False {
                w312 = T9 2 items=["START_STREAM", "PAUSE_STREAM", "STOP_STREAM"] ("uStreamState IN")
                n103 = call <vilib>:"MEPU-Acquisition-SetStreamState.vi"("hCamera IN"=w311, "uStreamState IN"=w312, "Error IN"=w310) -> ("hCamera OUT"=w309:u32, "Error OUT"=w308:errorcluster)  [unwired: 11 in]
              }
              frame True {
                w317 = T9 0 items=["START_STREAM", "PAUSE_STREAM", "STOP_STREAM"] ("uStreamState IN")
                n104 = call <vilib>:"MEPU-Acquisition-SetStreamState.vi"("hCamera IN"=w316, "uStreamState IN"=w317, "Error IN"=w315) -> ("hCamera OUT"=w313:u32, "Error OUT"=w314:errorcluster)  [unwired: 11 in]
              }
            }
          }
          event "Exposure Time (ms)": Value Change {
            w339 = T10 7 items=["FEATURE_BRIGHTNESS", "FEATURE_EXPOSURE", "FEATURE_SHARPNESS", "FEATURE_WHITE_BAL", "FEATURE_HUE", "FEATURE_SATURATION", "FEATURE_GAMMA", "FEATURE_SHUTTER", "FEATURE_GAIN", "FEATURE_IRIS", "FEATURE_FOCUS", "FEATURE_TEMPERATURE", "FEATURE_TRIGGER", "FEATURE_ZOOM", "FEATURE_PAN", "FEATURE_TILT", "FEATURE_OPT_FILTER", "FEATURE_GPIO", "FEATURE_FRAME_RATE", "FEATURE_ROI", "FEATURE_FLIP", "FEATURE_PIXEL_ADDRESSING", "FEATURE_PIXEL_FORMAT", "FEATURE_EXTENDED_SHUTTER", "FEATURE_AUTO_ROI", "FEATURE_LOOKUP_TABLE", "FEATURE_MEMORY_CHANNEL", "FEATURE_WHITE_SHADING", "FEATURE_ROTATE", "FEATURE_IMAGER_CLK_DIVISOR", "FEATURE_TRIG_WITH_CNTRLD_LIGHT", "FEATURE_MAX_PIXEL_SIZE"] ("uFeatureId IN")
            w353 = T9 2 items=["START_STREAM", "PAUSE_STREAM", "STOP_STREAM"] ("uStreamState IN")
            w359 = T11 1 items=["FEATURE_FLAG_PRESENCE                 0x00000001", "FEATURE_FLAG_MANUAL                     0x00000002", "FEATURE_FLAG_AUTO                         0x00000004", "FEATURE_FLAG_ONEPUSH                   0x00000008", "FEATURE_FLAG_OFF                            0x00000010", "FEATURE_FLAG_DESC_SUPPORTED    0x00000020", "FEATURE_FLAG_READ_ONLY               0x00000040"] ("uFlags IN")
            w360 = T10 7 items=["FEATURE_BRIGHTNESS", "FEATURE_EXPOSURE", "FEATURE_SHARPNESS", "FEATURE_WHITE_BAL", "FEATURE_HUE", "FEATURE_SATURATION", "FEATURE_GAMMA", "FEATURE_SHUTTER", "FEATURE_GAIN", "FEATURE_IRIS", "FEATURE_FOCUS", "FEATURE_TEMPERATURE", "FEATURE_TRIGGER", "FEATURE_ZOOM", "FEATURE_PAN", "FEATURE_TILT", "FEATURE_OPT_FILTER", "FEATURE_GPIO", "FEATURE_FRAME_RATE", "FEATURE_ROI", "FEATURE_FLIP", "FEATURE_PIXEL_ADDRESSING", "FEATURE_PIXEL_FORMAT", "FEATURE_EXTENDED_SHUTTER", "FEATURE_AUTO_ROI", "FEATURE_LOOKUP_TABLE", "FEATURE_MEMORY_CHANNEL", "FEATURE_WHITE_SHADING", "FEATURE_ROTATE", "FEATURE_IMAGER_CLK_DIVISOR", "FEATURE_TRIG_WITH_CNTRLD_LIGHT", "FEATURE_MAX_PIXEL_SIZE"] ("uFeatureId IN")
            n105 = event-data() -> ("NewVal"=w334:dbl)  [unwired: 1 in, 4 out]
            n106 = Divide(x=w334, y=1000.0) -> (x/y=w346:dbl)
            n107 = call <vilib>:"MEPU-Acquisition-SetStreamState.vi"("hCamera IN"=w349, "uStreamState IN"=w353, "Error IN"=w348) -> ("hCamera OUT"=w355:u32, "Error OUT"=w354:errorcluster)  [unwired: 11 in]
            n108 = To Double Precision Float(number=w346) -> (double precision float=w357:dbl)
            n109 = Build Array(w357) -> (w358:dbl[])
            n110 = call <vilib>:"MEPU-CameraFeatures-SetFeature.vi"("hCamera IN"=w355, "uFeatureId IN"=w360, "uFlags IN"=w359, "pParms IN"=w358, "Error IN"=w354) -> ("hCamera OUT"=w338:u32, "Error OUT"=w356:errorcluster)  [unwired: 8 in, 1 out]
            n111 = case shown="Error" w356 {
              tunnel: [w371 errorcluster {"status"=FALSE, "code"=0, "source"=""} ("Error OUT")] -> w335
              tunnel: w356 -> [w371 _]
              frame No Error {
              }
              frame Error {
                n112 = One Button Dialog(message="Ocurrio un error con shutter time") -> ()  [unwired: 1 in, 1 out]
              }
            }
            n113 = call <vilib>:"MEPU-CameraFeatures-GetFeature.vi"("hCamera IN"=w338, "uFeatureId IN"=w339, "Error IN"=w335) -> ("hCamera OUT"=w337:u32, "pParms OUT"=w340:dbl[], "Error OUT"=w336:errorcluster)  [unwired: 8 in, 2 out]
            n114 = Index Array(array=w340, index=0) -> (element=w343:dbl)
            n115 = case shown="True" w347 {
              tunnel: w336 -> [w364 w369]
              tunnel: [w362 w368] -> w350
              tunnel: [w363 w367] -> w351
              tunnel: w337 -> [w361 w366]
              frame False {
                w365 = T9 2 items=["START_STREAM", "PAUSE_STREAM", "STOP_STREAM"] ("uStreamState IN")
                n116 = call <vilib>:"MEPU-Acquisition-SetStreamState.vi"("hCamera IN"=w361, "uStreamState IN"=w365, "Error IN"=w364) -> ("hCamera OUT"=w363:u32, "Error OUT"=w362:errorcluster)  [unwired: 11 in]
              }
              frame True {
                w370 = T9 0 items=["START_STREAM", "PAUSE_STREAM", "STOP_STREAM"] ("uStreamState IN")
                n117 = call <vilib>:"MEPU-Acquisition-SetStreamState.vi"("hCamera IN"=w366, "uStreamState IN"=w370, "Error IN"=w369) -> ("hCamera OUT"=w367:u32, "Error OUT"=w368:errorcluster)  [unwired: 11 in]
              }
            }
            n118 = Multiply(x=w343, y=1000) -> (x*y=w321:dbl)
            n119 = property on="Exposure Time (ms)" class="Slide (strict)"("Value"=w321) -> ()  [unwired: 2 in, 2 out]
            n120 = Divide(x=w321, y=sgl 1000.0) -> (x/y=w326:dbl)
            n121 = call "Restart DAQ.vi"("Min Value"=w324, "tiempo (s)"=w326, "Max Value"=w325, "error IN"=w327, "Fs (S/s)"=w322, "Physical Channel"=w323, "task IN"=w328) -> ("error OUT"=w330:errorcluster, "# samples"=w329:u32, "task OUT"=w331:refnum<k21>)  [unwired: 2 in]
          }
          event "Physical Channel", "Minimum Value", "Maximum Value", "DAQ Fs (S/s)": Value Change {
            n122 = event-data() -> ()  [unwired: 1 in, 5 out]
            n123 = call "Restart DAQ.vi"("Min Value"=w376, "tiempo (s)"=w379, "Max Value"=w375, "error IN"=w382, "Fs (S/s)"=w374, "Physical Channel"=w380, "task IN"=w383) -> ("error OUT"=w378:errorcluster, "# samples"=w377:u32, "task OUT"=w381:refnum<k21>)  [unwired: 2 in]
          }
          event "Gain": Value Change {
            w400 = T10 8 items=["FEATURE_BRIGHTNESS", "FEATURE_EXPOSURE", "FEATURE_SHARPNESS", "FEATURE_WHITE_BAL", "FEATURE_HUE", "FEATURE_SATURATION", "FEATURE_GAMMA", "FEATURE_SHUTTER", "FEATURE_GAIN", "FEATURE_IRIS", "FEATURE_FOCUS", "FEATURE_TEMPERATURE", "FEATURE_TRIGGER", "FEATURE_ZOOM", "FEATURE_PAN", "FEATURE_TILT", "FEATURE_OPT_FILTER", "FEATURE_GPIO", "FEATURE_FRAME_RATE", "FEATURE_ROI", "FEATURE_FLIP", "FEATURE_PIXEL_ADDRESSING", "FEATURE_PIXEL_FORMAT", "FEATURE_EXTENDED_SHUTTER", "FEATURE_AUTO_ROI", "FEATURE_LOOKUP_TABLE", "FEATURE_MEMORY_CHANNEL", "FEATURE_WHITE_SHADING", "FEATURE_ROTATE", "FEATURE_IMAGER_CLK_DIVISOR", "FEATURE_TRIG_WITH_CNTRLD_LIGHT", "FEATURE_MAX_PIXEL_SIZE"] ("uFeatureId IN")
            w410 = T9 2 items=["START_STREAM", "PAUSE_STREAM", "STOP_STREAM"] ("uStreamState IN")
            w416 = T11 1 items=["FEATURE_FLAG_PRESENCE                 0x00000001", "FEATURE_FLAG_MANUAL                     0x00000002", "FEATURE_FLAG_AUTO                         0x00000004", "FEATURE_FLAG_ONEPUSH                   0x00000008", "FEATURE_FLAG_OFF                            0x00000010", "FEATURE_FLAG_DESC_SUPPORTED    0x00000020", "FEATURE_FLAG_READ_ONLY               0x00000040"] ("uFlags IN")
            w417 = T10 8 items=["FEATURE_BRIGHTNESS", "FEATURE_EXPOSURE", "FEATURE_SHARPNESS", "FEATURE_WHITE_BAL", "FEATURE_HUE", "FEATURE_SATURATION", "FEATURE_GAMMA", "FEATURE_SHUTTER", "FEATURE_GAIN", "FEATURE_IRIS", "FEATURE_FOCUS", "FEATURE_TEMPERATURE", "FEATURE_TRIGGER", "FEATURE_ZOOM", "FEATURE_PAN", "FEATURE_TILT", "FEATURE_OPT_FILTER", "FEATURE_GPIO", "FEATURE_FRAME_RATE", "FEATURE_ROI", "FEATURE_FLIP", "FEATURE_PIXEL_ADDRESSING", "FEATURE_PIXEL_FORMAT", "FEATURE_EXTENDED_SHUTTER", "FEATURE_AUTO_ROI", "FEATURE_LOOKUP_TABLE", "FEATURE_MEMORY_CHANNEL", "FEATURE_WHITE_SHADING", "FEATURE_ROTATE", "FEATURE_IMAGER_CLK_DIVISOR", "FEATURE_TRIG_WITH_CNTRLD_LIGHT", "FEATURE_MAX_PIXEL_SIZE"] ("uFeatureId IN")
            n124 = event-data() -> ("NewVal"=w394:dbl)  [unwired: 1 in, 4 out]
            n125 = To Double Precision Float(number=w394) -> (double precision float=w414:dbl)
            n126 = call <vilib>:"MEPU-Acquisition-SetStreamState.vi"("hCamera IN"=w406, "uStreamState IN"=w410, "Error IN"=w405) -> ("hCamera OUT"=w412:u32, "Error OUT"=w411:errorcluster)  [unwired: 11 in]
            n127 = Build Array(w414) -> (w415:dbl[])
            n128 = call <vilib>:"MEPU-CameraFeatures-SetFeature.vi"("hCamera IN"=w412, "uFeatureId IN"=w417, "uFlags IN"=w416, "pParms IN"=w415, "Error IN"=w411) -> ("hCamera OUT"=w399:u32, "Error OUT"=w413:errorcluster)  [unwired: 8 in, 1 out]
            n129 = case shown="Error" w413 {
              tunnel: [w428 errorcluster {"status"=FALSE, "code"=0, "source"=""} ("Error OUT")] -> w396
              tunnel: w413 -> [w428 _]
              frame No Error {
              }
              frame Error {
                n130 = One Button Dialog(message="Ocurrio un error con Gain") -> ()  [unwired: 1 in, 1 out]
              }
            }
            n131 = call <vilib>:"MEPU-CameraFeatures-GetFeature.vi"("hCamera IN"=w399, "uFeatureId IN"=w400, "Error IN"=w396) -> ("hCamera OUT"=w398:u32, "pParms OUT"=w401:dbl[], "Error OUT"=w397:errorcluster)  [unwired: 8 in, 2 out]
            n132 = case shown="True" w404 {
              tunnel: w397 -> [w421 w426]
              tunnel: [w419 w425] -> w407
              tunnel: [w420 w424] -> w408
              tunnel: w398 -> [w418 w423]
              frame False {
                w422 = T9 2 items=["START_STREAM", "PAUSE_STREAM", "STOP_STREAM"] ("uStreamState IN")
                n133 = call <vilib>:"MEPU-Acquisition-SetStreamState.vi"("hCamera IN"=w418, "uStreamState IN"=w422, "Error IN"=w421) -> ("hCamera OUT"=w420:u32, "Error OUT"=w419:errorcluster)  [unwired: 11 in]
              }
              frame True {
                w427 = T9 0 items=["START_STREAM", "PAUSE_STREAM", "STOP_STREAM"] ("uStreamState IN")
                n134 = call <vilib>:"MEPU-Acquisition-SetStreamState.vi"("hCamera IN"=w423, "uStreamState IN"=w427, "Error IN"=w426) -> ("hCamera OUT"=w424:u32, "Error OUT"=w425:errorcluster)  [unwired: 11 in]
              }
            }
            n135 = Index Array(array=w401, index=0) -> (element=w393:dbl)
            n136 = property on="Gain" class="Slide (strict)"("Value"=w393) -> ()  [unwired: 2 in, 2 out]
          }
        }
        n137 = call <vilib>:"Simple Error Handler.vi"("error in (no error)"=w87) -> ("error out"=w91:errorcluster)  [unwired: 1 in, 7 out]
        n138 = call <vilib>:"Simple Error Handler.vi"("error in (no error)"=w84) -> ("error out"=w83:errorcluster)  [unwired: 1 in, 7 out]
        n139 = case shown="Error" w91 {
          selector: w91 -> [w105 _]
          tunnel: [w105 errorcluster {"status"=FALSE, "code"=0, "source"=""} ("error IO")] -> w64
          tunnel: [FALSE ("T button?") w107] -> w90
          frame No Error {
          }
          frame Error {
            n140 = Two Button Dialog(message="An error was detected.\nDo you wish to continue execution?", 1:"Stop" ("F button name (\"Cancel\")"), 2:"Continue" ("T button name (\"OK\")")) -> (T button?=w108:bool)
            n141 = Not(x=w108) -> (.not. x?=w107:bool)
          }
        }
        n142 = case shown="Error" w83 {
          selector: w83 -> [w97 _]
          tunnel: [w97 errorcluster {"status"=FALSE, "code"=0, "source"=""} ("error IO")] -> w72
          tunnel: [FALSE ("T button?") w99] -> w80
          frame No Error {
          }
          frame Error {
            n143 = Two Button Dialog(message="An error was detected.\nDo you wish to continue execution?", 1:"Stop" ("F button name (\"Cancel\")"), 2:"Continue" ("T button name (\"OK\")")) -> (T button?=w100:bool)
            n144 = Not(x=w100) -> (.not. x?=w99:bool)
          }
        }
        n145 = property on="Stop App" class="Bool (strict)"() -> ("Value"=w82:bool)  [unwired: 2 in, 2 out]
        n146 = property on="Stop App" class="Bool (strict)"() -> ("Value"=w88:bool)  [unwired: 2 in, 2 out]
        n147 = Or(x=w80, y=w82) -> (x .or. y?=w69:bool)
        n148 = Or(x=w90, y=w88) -> (x .or. y?=w70:bool)
        n149 = Or(x=w70, y=w69) -> (x .or. y?=w81:bool)
      }
      n150 = call <vilib>:"MEPU-Initialization-Uninitialize.vi"("hCamera IN"=w46, "Error IN"=w30) -> ()  [unwired: 13 in, 1 out]
      n151 = call <vilib>:"DAQmx Clear Task.vi"("task in"=w10, "error in"=w9) -> ("error out"=w12:errorcluster)  [unwired: 13 in]
      n152 = call <vilib>:"Simple Error Handler.vi"("type of dialog (OK msg:1)"=w11, "error in (no error)"=w12) -> ()  [unwired: 3 in, 5 out]
    }
  }
